vi "azcamtool.vi"() -> ()   [LabVIEW 2014]
doc: "AzCamTool"
uses:
  globals/AzCamGlobals.vi
  globals/DetectorGlobals.vi
panel:
  in  "Image Type":u16(ring) items=["zero", "object", "flat", "dark", "Fe55"]
  in  "Exposure Time":dbl=1.0 min=0.0 format="%<%S%3u>t"
  out "Image Filename":string
  out "StatusBar":string
  in  "TestImage":bool=TRUE caption="Test Image"
  in  "Image Title":string
  out "rowbin":u32=1 min=1 max=99 step=1
  out "colbin":u32=1 min=1 max=99 step=1
  out "progress":dbl(slide) scale=0.0..100.0 scale format="%.1e"
  out "CamTemp":sgl=-999.9 format="%.1f"
  out "DewTemp":sgl=-999.9 format="%.1f"
  out "SequenceCount":string caption="Seq. Count"
  out "Current Exposure Time":dbl caption="Exposure Time" min=0.0 format="%<%S%3u>t"
  out "ImageTypeName":string caption="ImageType"
  in  "Abort":bool
  in  "Reset":bool
  in  "Pause":bool
  in  "Resume":bool
  in  "Readout":bool
  out "CurrentImageTitle":string caption="ImageTitle"
  in  "Expose":bool
  in  "Sequence":bool
  in  "Num Seq.":u16=1 min=1 step=1
  in  "Detector":bool
  in  "FilenameBut":bool caption="Filename"
  in  "Preferences":bool
  out "Test Image":bool
  # "Control"
  # "Status"
  # "Binning"
  # "Exposure Status"
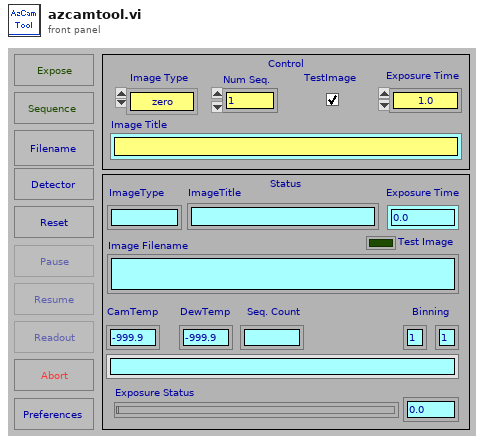
[diagram p1: front panel]
types:
  T1 = enum16{"Standard", "Buffered", "CRLF", "Immediate"}
  T2 = enum16{"Start", "Stop", "Abort", "Pause", "SetExposureTime", "GetExposureTimeRemaining", "Resume", "Readout", "GetExposureTime", "GetTotalPixels", "GetPixelsRemaining"}
  T3 = enum16{"Start", "Stop", "Abort", "Pause", "SetExposureTime", "GetExposureTimeRemaining", "Resume", "Readout", "GetExposureTime"}
  T4 = enum16{"Start", "Stop", "Abort", "Pause", "SetExposureTime", "GetExposureTimeRemaining", "Resume"}
  T5 = enum16{"Start", "Stop", "Abort", "Pause", "SetExposureTime", "GetExposureTimeRemaining", "Resume", "Readout"}
  T6 = enum32{"invalid app kind", "Development System", "Run Time System", "Student Edition", "Embedded LabVIEW", "Evaluation", "Custom"}
  T7 = enum32{"invalid OS target", "Mac OS", "Windows 3.1", "Windows 95/NT", "Solaris 1", "Solaris 2", "HP-UX", "PowerMAX", "Linux", "Irix", "Rhapsody", "BeOS", "AIX", "OSF1", "VxWorks", "PharLap", "Carbon", "RTX", "Windows x64", "Linux x64", "Mac OS X x64"}
  T8 = enum8{"Enabled", "Disabled", "Disabled and Grayed Out"}
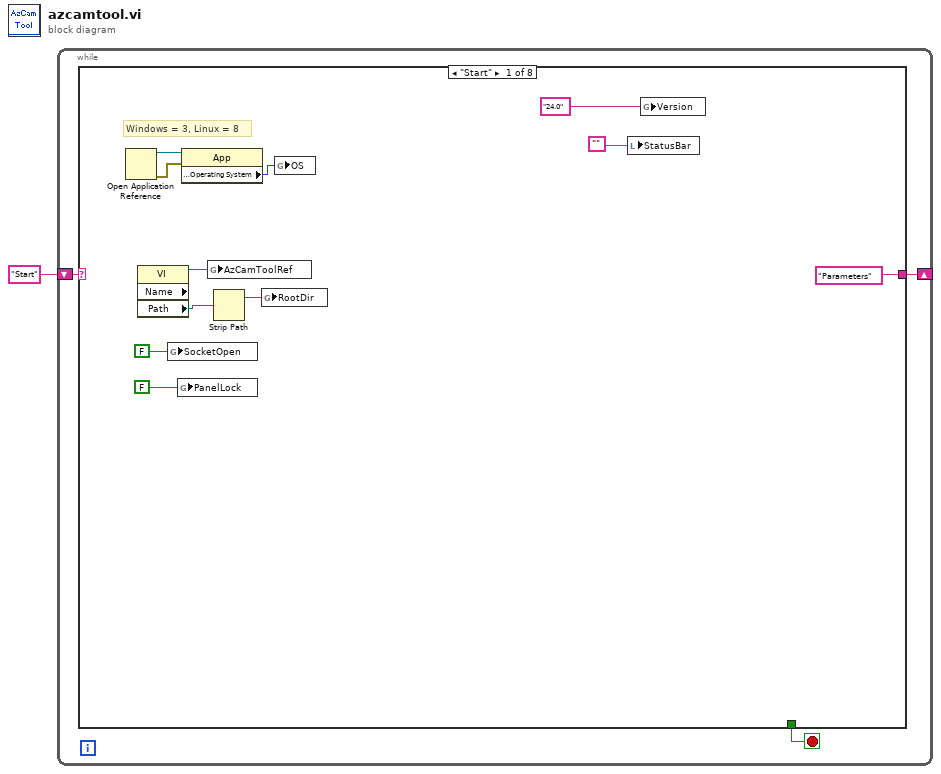
[diagram p0: block diagram]
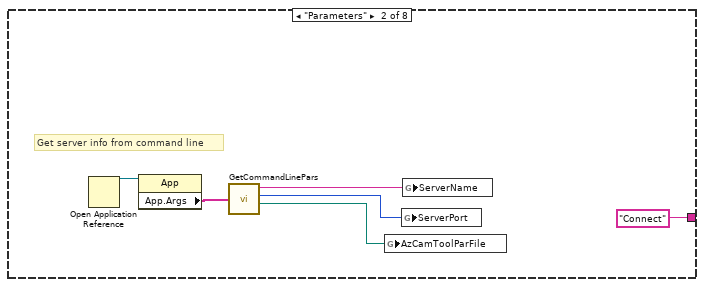
[diagram p2: hidden frame]
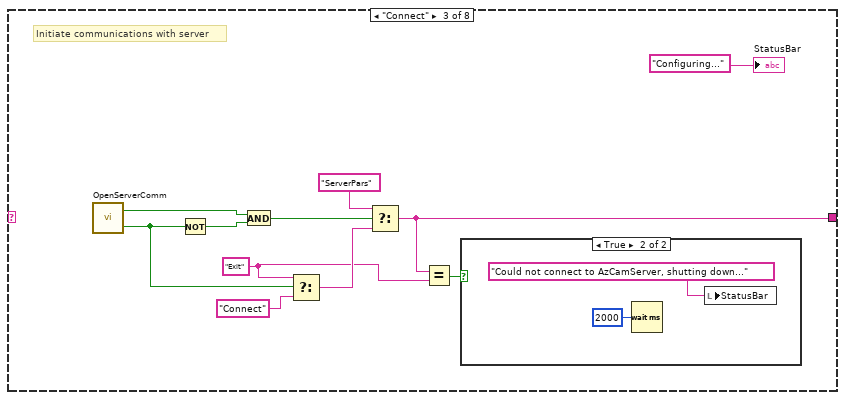
[diagram p3: hidden frame]
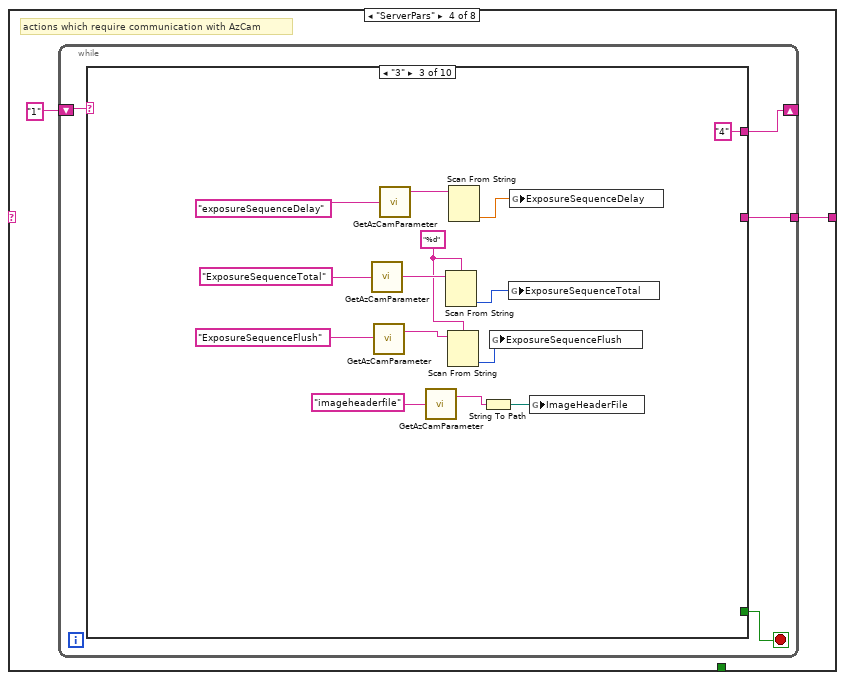
[diagram p5: hidden frame]
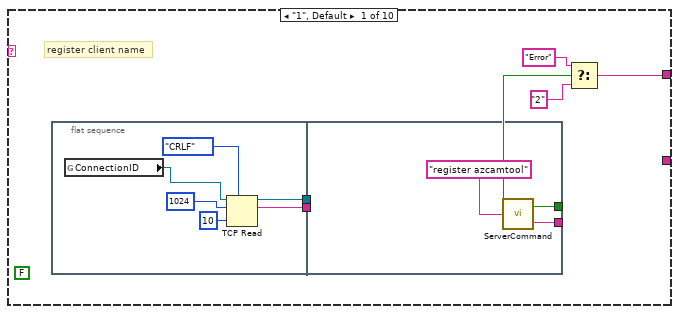
[diagram p6: hidden frame]
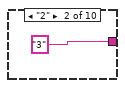
[diagram p7: hidden frame]
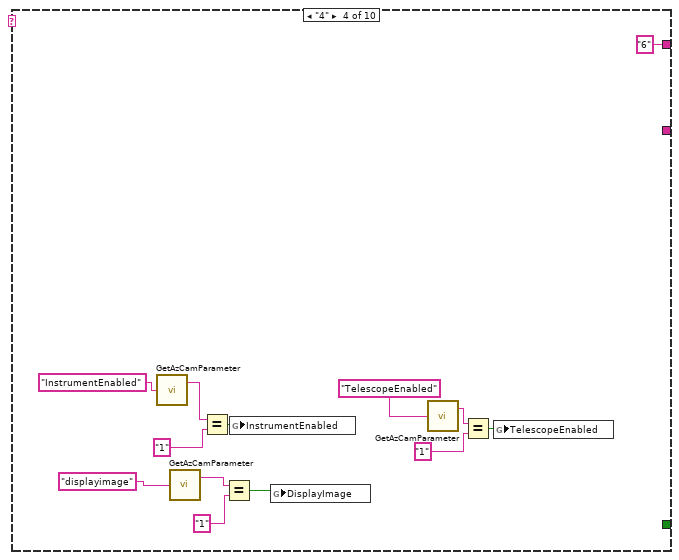
[diagram p8: hidden frame]
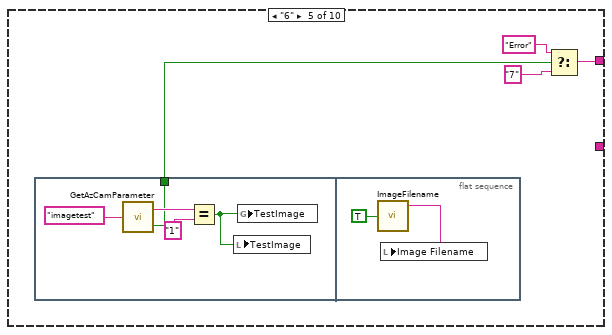
[diagram p9: hidden frame]
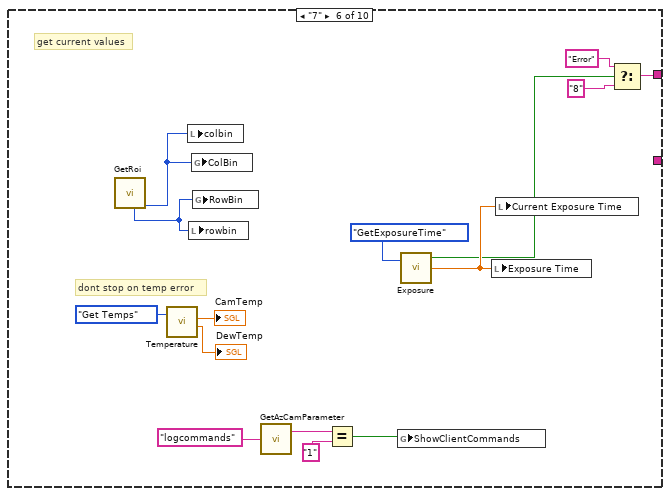
[diagram p10: hidden frame]
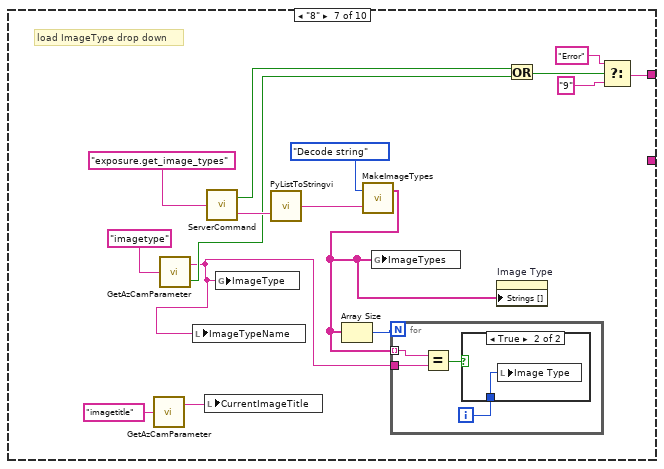
[diagram p11: hidden frame]
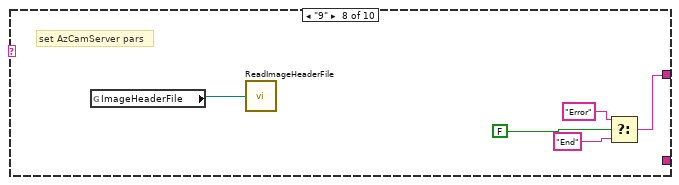
[diagram p13: hidden frame]
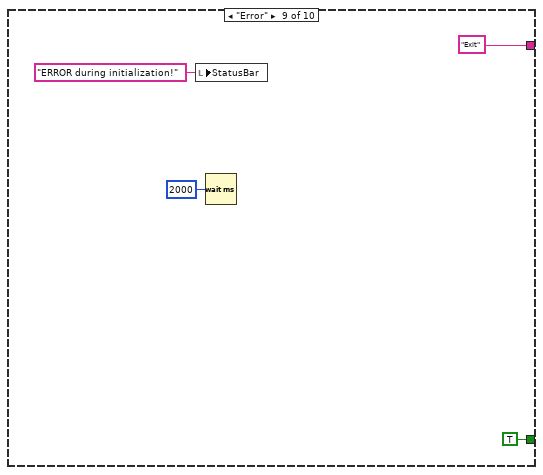
[diagram p14: hidden frame]
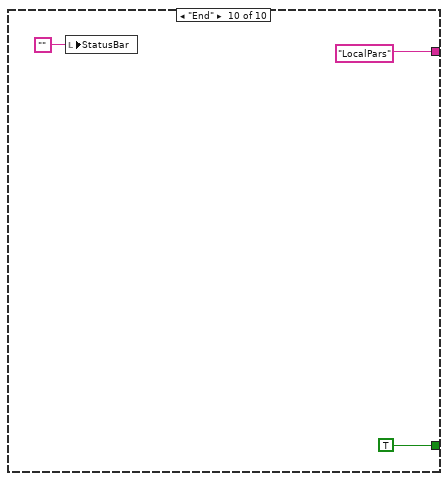
[diagram p15: hidden frame]
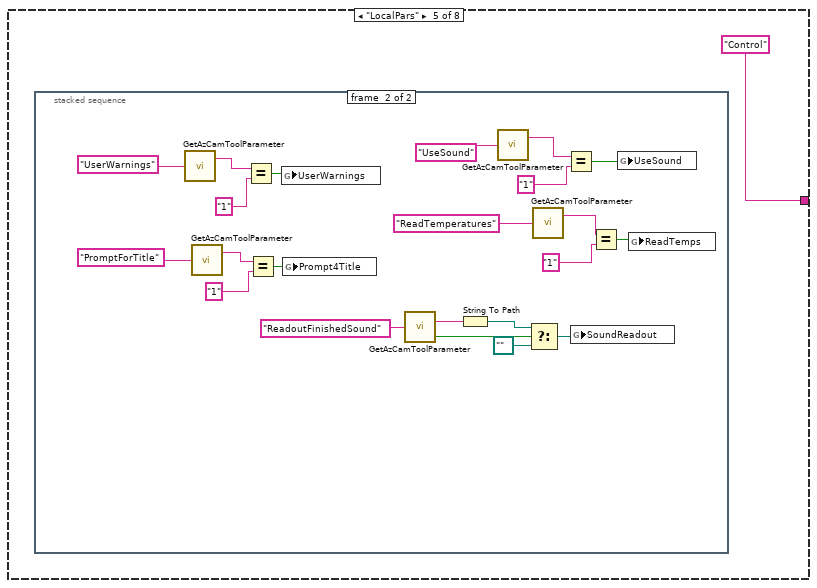
[diagram p16: hidden frame]
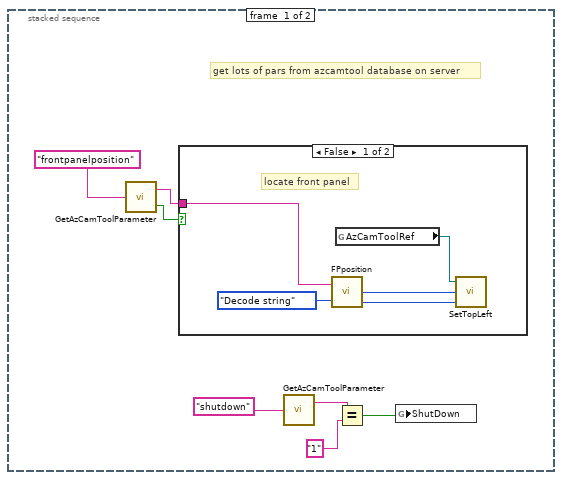
[diagram p17: hidden frame]
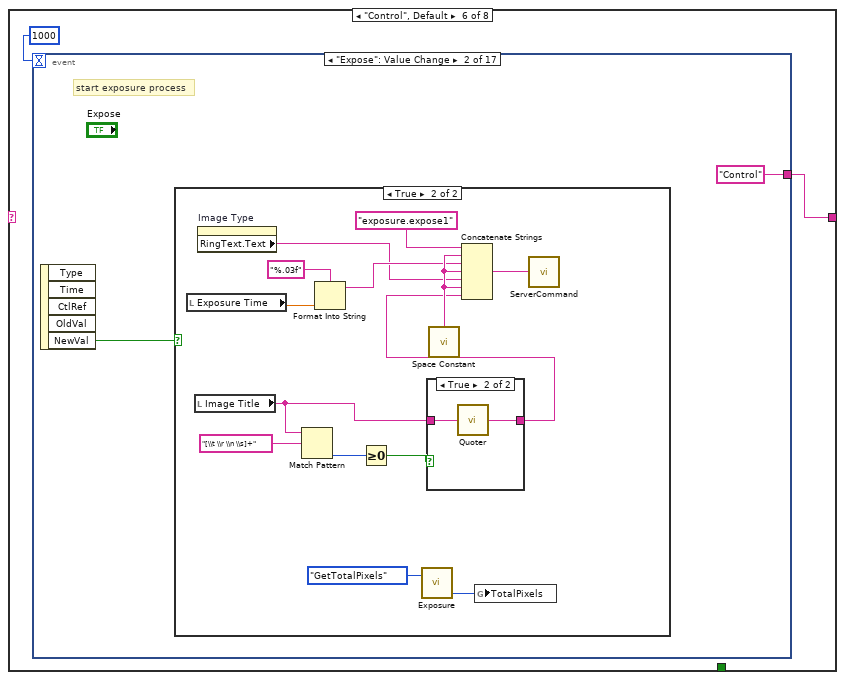
[diagram p19: hidden frame]
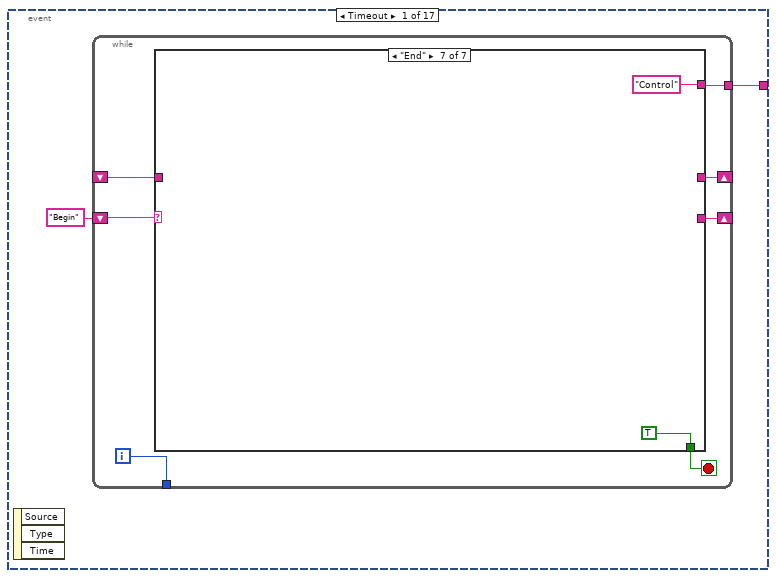
[diagram p20: hidden frame]
diagram:
  n1 = while {
    shift-right: [w2] -> _
    shift-left: "Start" ("Command") -> [w3]
    stop <- w4 stop-if-true
    n2 = case shown="\"Start\"" w3 {
      tunnel: [_ _ _ _ _ _ TRUE TRUE] -> w4
      tunnel: ["Parameters" "Connect" ("f") w24 w36 "Control" w179 _ _] -> w2
      frame "Start" {
        # "Windows = 3, Linux = 8"
        n3 = Open Application Reference() -> (0:w14:errorcluster, 3:w15:refnum<vi>)  [unwired: 4 in]
        n4 = property class="VI" props=["Name", "Path"]() -> (reference out=w6:refnum<vi>, "Path"=w10:path)  [unwired: 2 in, 2 out]
        n5 = global write "AzCamGlobals.vi" "SocketOpen"(FALSE ("SocketOpen")) -> ()
        n6 = global write "AzCamGlobals.vi" "PanelLock"(FALSE ("LockFlag")) -> ()
        n7 = property class="App"(reference=w15, error in=w14) -> ("Application:Target:Operating System"=w12:T7)  [unwired: 2 out]
        n8 = global write "AzCamGlobals.vi" "AzCamToolRef"(w6) -> ()
        n9 = Strip Path(path=w10) -> (stripped path=w8:path)  [unwired: 1 out]
        n10 = global write "AzCamGlobals.vi" "RootDir"(w8) -> ()
        n11 = global write "AzCamGlobals.vi" "OS"(w12) -> ()
        n12 = local write "StatusBar"("") -> ()
        n13 = global write "AzCamGlobals.vi" "Version"("24.0" ("Version Date")) -> ()
      }
      frame "Parameters" {
        # "Get server info from command line"
        n14 = Open Application Reference() -> (3:w19:refnum<vi>)  [unwired: 4 in, 1 out]
        n15 = property class="App"(reference=w19) -> ("App.Args"=w20:string[])  [unwired: 1 in, 2 out]
        n16 = call "GetCommandLinePars.vi"("Command line array"=w20) -> ("Server"=w18:string, "Port"=w17:i32, "AzCamToolParFile"=w16:path)  [unwired: 1 out]
        n17 = global write "AzCamGlobals.vi" "AzCamToolParFile"(w16) -> ()
        n18 = global write "AzCamGlobals.vi" "ServerPort"(w17) -> ()
        n19 = global write "AzCamGlobals.vi" "ServerName"(w18) -> ()
      }
      frame "Connect" {
        w23 = "Exit" ("f")
        # "Initiate communications with server"
        n20 = call "OpenServerComm.vi"() -> ("Connected"=w31:bool, "Quitted"=w25:bool)  [unwired: 1 in]
        n21 = Not(x=w25) -> (.not. x?=w30:bool)
        n22 = And(x=w31, y=w30) -> (x .and. y?=w32:bool)
        n23 = Select(t=w23, s=w25, f="Connect") -> (s? t:f=w27:string)
        n24 = Select(t="ServerPars" ("f"), s=w32, f=w27) -> (s? t:f=w24:string)
        n25 = Equal?(x=w24, y=w23) -> (x = y?=w22:bool)
        n26 = case shown="True" w22 {
          frame False {
          }
          frame True {
            n27 = Wait (ms)(milliseconds to wait=u32 2000) -> ()  [unwired: 1 out]
            n28 = local write "StatusBar"("Could not connect to AzCamServer, shutting down..." ("StatusBar")) -> ()
          }
        }
        "StatusBar" <- "Configuring..." ("Messages")
      }
      frame "ServerPars" {
        # "actions which require communication with AzCam"
        n29 = while {
          tunnel: [w38] -> w36
          shift-right: [w39] -> _
          shift-left: "1" ("key") -> [w40]
          stop <- w37 stop-if-true
          n30 = case shown="\"3\"" w40 {
            tunnel: [w44 "3" ("key") "4" ("key") "6" ("key") w85 w104 w116 w133 _ _] -> w39
            tunnel: [_ _ _ _ _ _ _ _ "Exit" "LocalPars"] -> w38
            tunnel: [_ _ _ _ _ _ _ _ TRUE TRUE] -> w37
            frame "1", Default {
              (unwired) FALSE
              # "register client name"
              n31 = flat-sequence {
                tunnel: [w49] -> w42
                tunnel: [w48] -> w41
                tunnel: [w54] -> _
                tunnel: [w53] -> w43
                tunnel: w42 -> [_]
                tunnel: w41 -> [_]
                frame #0 {
                  n32 = global read "AzCamGlobals.vi" "ConnectionID"() -> (w47:refnum<k5>)
                  n33 = TCP Read(connection ID=w47, bytes to read=1024, 7:T1."CRLF" ("mode (standard)"), 9:10 ("timeout ms (25000)")) -> (connection ID out=w48:refnum<k5>, data out=w49:string)  [unwired: 1 in, 1 out]
                }
                frame #1 {
                  n34 = call "ServerCommand.vi"("Command"="register azcamtool") -> ("Error"=w53:bool, "Reply"=w54:string)
                }
              }
              n35 = Select(t="Error" ("key"), s=w43, f="2" ("key")) -> (s? t:f=w44:string)
            }
            frame "2" {
            }
            frame "3" {
              w65 = "%d" ("format string")
              n36 = call "GetAzCamParameter.vi"("Parameter"="ExposureSequenceTotal") -> ("Value"=w69:string)  [unwired: 1 out]
              n37 = call "GetAzCamParameter.vi"("Parameter"="ExposureSequenceFlush") -> ("Value"=w60:string)  [unwired: 1 out]
              n38 = call "GetAzCamParameter.vi"("Parameter"="exposureSequenceDelay") -> ("Value"=w67:string)  [unwired: 1 out]
              n39 = call "GetAzCamParameter.vi"("Parameter"="imageheaderfile" ("key")) -> ("Value"=w59:string)  [unwired: 1 out]
              n40 = Scan From String(format string=w65, input string=w69) -> (output 1=w63:i32)  [unwired: 3 in, 3 out]
              n41 = Scan From String(format string=w65, input string=w60) -> (output 1=w64:i32)  [unwired: 3 in, 3 out]
              n42 = Scan From String(input string=w67) -> (output 1=w62:dbl)  [unwired: 4 in, 3 out]
              n43 = String To Path(string=w59) -> (path=w61:path)
              n44 = global write "AzCamGlobals.vi" "ExposureSequenceFlush"(w64) -> ()
              n45 = global write "AzCamGlobals.vi" "ExposureSequenceTotal"(w63) -> ()
              n46 = global write "AzCamGlobals.vi" "ExposureSequenceDelay"(w62) -> ()
              n47 = global write "AzCamGlobals.vi" "ImageHeaderFile"(w61) -> ()
            }
            frame "4" {
              n48 = call "GetAzCamParameter.vi"("Parameter"="InstrumentEnabled" ("key")) -> ("Value"=w71:string)  [unwired: 1 out]
              n49 = call "GetAzCamParameter.vi"("Parameter"="displayimage" ("key")) -> ("Value"=w74:string)  [unwired: 1 out]
              n50 = Equal?(x=w71, y="1") -> (x = y?=w79:bool)
              n51 = Equal?(x=w74, y="1") -> (x = y?=w78:bool)
              n52 = global write "AzCamGlobals.vi" "InstrumentEnabled"(w79) -> ()
              n53 = global write "AzCamGlobals.vi" "DisplayImage"(w78) -> ()
              n54 = call "GetAzCamParameter.vi"("Parameter"="TelescopeEnabled" ("key")) -> ("Value"=w75:string)  [unwired: 1 out]
              n55 = Equal?(x=w75, y="1") -> (x = y?=w82:bool)
              n56 = global write "AzCamGlobals.vi" "TelescopeEnabled"(w82) -> ()
            }
            frame "6" {
              n57 = flat-sequence {
                tunnel: [w88] -> w84
                frame #0 {
                  n58 = call "GetAzCamParameter.vi"("Parameter"="imagetest") -> ("Error"=w88:bool, "Value"=w89:string)
                  n59 = Equal?(x=w89, y="1") -> (x = y?=w92:bool)
                  n60 = local write "TestImage"(w92) -> ()
                  n61 = global write "AzCamGlobals.vi" "TestImage"(w92) -> ()
                }
                frame #1 {
                  n62 = call "ImageFilename.vi"("Immediate"=TRUE) -> ("Output Image Filename"=w94:string)  [unwired: 2 out]
                  n63 = local write "Image Filename"(w94) -> ()
                }
              }
              n64 = Select(t="Error" ("key"), s=w84, f="7" ("key")) -> (s? t:f=w85:string)
            }
            frame "7" {
              # "dont stop on temp error"
              # "get current values"
              n65 = call "GetRoi.vi"() -> ("RowBin"=w108:i32, "ColBin"=w109:i32)  [unwired: 1 in, 4 out]
              n66 = call "Temperature.vi"("Action"=enum16{"Set Celsius", "Get Temps"}."Get Temps") -> ("Output2"=→"DewTemp":sgl, "Output1"=→"CamTemp":sgl)  [unwired: 1 in, 3 out]
              n67 = local write "colbin"(w109) -> ()
              n68 = local write "rowbin"(w108) -> ()
              n69 = global write "DetectorGlobals.vi" "ColBin"(w109) -> ()
              n70 = global write "DetectorGlobals.vi" "RowBin"(w108) -> ()
              n71 = call "GetAzCamParameter.vi"("Parameter"="logcommands") -> ("Value"=w96:string)  [unwired: 1 out]
              n72 = Equal?(x=w96, y="1") -> (x = y?=w95:bool)
              n73 = global write "AzCamGlobals.vi" "ShowClientCommands"(w95) -> ()
              n74 = call "Exposure.vi"("Command"=T2."GetExposureTime") -> ("Error"=w99:bool, "float"=w100:dbl)  [unwired: 1 in, 1 out]
              n75 = local write "Exposure Time"(w100) -> ()
              n76 = local write "Current Exposure Time"(w100) -> ()
              n77 = Select(t="Error" ("key"), s=w99, f="8" ("key")) -> (s? t:f=w104:string)
            }
            frame "8" {
              # "load ImageType drop down"
              n78 = call "GetAzCamParameter.vi"("Parameter"="imagetitle") -> ("Value"=w110:string)  [unwired: 1 out]
              n79 = call "GetAzCamParameter.vi"("Parameter"="imagetype") -> ("Error"=w113:bool, "Value"=w112:string)
              n80 = local write "ImageTypeName"(w112) -> ()
              n81 = local write "CurrentImageTitle"(w110) -> ()
              n82 = call "ServerCommand.vi"("Command"="exposure.get_image_types") -> ("Error"=w114:bool, "Reply"=w123:string)
              n83 = global write "AzCamGlobals.vi" "ImageType"(w112) -> ()
              n84 = call "PyListToStringvi.vi"("PythonList"=w123) -> ("String"=w122:string)
              n85 = call "MakeImageTypes.vi"("String In"=w122, "Action"=enum16{"Make string", "Decode string"}."Decode string") -> ("ImageTypes"=w120:string[])  [unwired: 1 out]
              n86 = Array Size(array=w120) -> (size(s)=w121:i32)
              n87 = global write "AzCamGlobals.vi" "ImageTypes"(w120) -> ()
              n88 = for {
                N: w121 -> [_]
                tunnel: w120 -> [w129] mode=indexing
                tunnel: w112 -> [w128]
                i -> [w126]
                n89 = Equal?(x=w129, y=w128) -> (x = y?=w127:bool)
                n90 = case shown="True" w127 {
                  tunnel: w126 -> [_ w130]
                  frame False {
                  }
                  frame True {
                    n91 = local write "Image Type"(w130) -> ()
                  }
                }
              }
              n92 = property on="Image Type" class="Ring (strict)"("Strings []"=w120) -> ()  [unwired: 2 in, 2 out]
              n93 = Or(x=w114, y=w113) -> (x .or. y?=w115:bool)
              n94 = Select(t="Error" ("key"), s=w115, f="9" ("key")) -> (s? t:f=w116:string)
            }
            frame "9" {
              # "set AzCamServer pars"
              n95 = global read "AzCamGlobals.vi" "ImageHeaderFile"() -> (w132:path)
              n96 = call "ReadImageHeaderFile.vi"("ImageHeaderFile"=w132) -> ()  [unwired: 1 in]
              n97 = Select(t="Error" ("key"), s=FALSE, f="End" ("key")) -> (s? t:f=w133:string)
            }
            frame "Error" {
              n98 = local write "StatusBar"("ERROR during initialization!" ("StatusBar")) -> ()
              n99 = Wait (ms)(milliseconds to wait=u32 2000) -> ()  [unwired: 1 out]
            }
            frame "End" {
              n100 = local write "StatusBar"("") -> ()
            }
          }
        }
      }
      frame "LocalPars" {
        n101 = stacked-sequence {
          frame #0 {
            # "get lots of pars from azcamtool database on server"
            n102 = call "GetAzCamToolParameter.vi"("Parameter"="frontpanelposition" ("key")) -> ("Error"=w149:bool, "Value"=w150:string)
            n103 = case shown="False" w149 {
              tunnel: w150 -> [w151 _]
              frame False {
                # "locate front panel"
                n104 = call "FPposition.vi"("String In"=w151, "Action"=enum16{"Make string", "Decode string"}."Decode string") -> ("top"=w153:i32, "left"=w152:i32)  [unwired: 1 out]
                n105 = global read "AzCamGlobals.vi" "AzCamToolRef"() -> (w155:refnum<vi>)
                n106 = call "SetTopLeft.vi"("left"=w152, "top"=w153, "VI Ref"=w155) -> ()
              }
              frame True {
              }
            }
            n107 = call "GetAzCamToolParameter.vi"("Parameter"="shutdown" ("key")) -> ("Value"=w144:string)  [unwired: 1 out]
            n108 = Equal?(x=w144, y="1") -> (x = y?=w147:bool)
            n109 = global write "AzCamGlobals.vi" "ShutDown"(w147) -> ()
          }
          frame #1 {
            n110 = call "GetAzCamToolParameter.vi"("Parameter"="UserWarnings" ("key")) -> ("Value"=w158:string)  [unwired: 1 out]
            n111 = call "GetAzCamToolParameter.vi"("Parameter"="PromptForTitle" ("key")) -> ("Value"=w159:string)  [unwired: 1 out]
            n112 = Equal?(x=w158, y="1") -> (x = y?=w176:bool)
            n113 = Equal?(x=w159, y="1") -> (x = y?=w174:bool)
            n114 = global write "AzCamGlobals.vi" "UserWarnings"(w176) -> ()
            n115 = global write "AzCamGlobals.vi" "Prompt4Title"(w174) -> ()
            n116 = call "GetAzCamToolParameter.vi"("Parameter"="ReadoutFinishedSound" ("key")) -> ("Error"=w156:bool, "Value"=w160:string)
            n117 = String To Path(string=w160) -> (path=w168:path)
            n118 = call "GetAzCamToolParameter.vi"("Parameter"="UseSound" ("key")) -> ("Value"=w177:string)  [unwired: 1 out]
            n119 = Select(t=w168, s=w156, f=path "") -> (s? t:f=w170:path)
            n120 = call "GetAzCamToolParameter.vi"("Parameter"="ReadTemperatures" ("key")) -> ("Value"=w165:string)  [unwired: 1 out]
            n121 = Equal?(x=w177, y="1") -> (x = y?=w171:bool)
            n122 = global write "AzCamGlobals.vi" "SoundReadout"(w170) -> ()
            n123 = Equal?(x=w165, y="1") -> (x = y?=w167:bool)
            n124 = global write "AzCamGlobals.vi" "UseSound"(w171) -> ()
            n125 = global write "AzCamGlobals.vi" "ReadTemps"(w167) -> ()
          }
        }
      }
      frame "Control", Default {
        n126 = event shown="[1] \"Expose\": Value Change" {
          selector: _ -> [_ _ _ _ _ _ _ _ _ _ _ _ _ _ _ _ _]
          dyn-events: _ -> [_ _ _ _ _ _ _ _ _ _ _ _ _ _ _ _ _]
          timeout: 1000 -> [_ _ _ _ _ _ _ _ _ _ _ _ _ _ _ _ _]
          tunnel: [w181 "Control" ("Command") "Control" ("Command") _ _ _ _ _ _ _ _ _ _ _ _ "Exit" ("Command") w408] -> w179
          event Timeout {
            n127 = event-data() -> ()  [unwired: 1 in, 3 out]
            n128 = while {
              shift-right: [w187] -> _
              shift-left: "Begin" -> [w188]
              tunnel: [w186] -> w181
              tunnel: [w185] -> _
              shift-right: [w184] -> _
              shift-left: _ -> [w183]
              i -> [w185]
              stop <- w182 stop-if-true
              n129 = case shown="\"End\"" w188 {
                tunnel: [w191 "Pars" "TimeSync" "CheckExposing" w249 "End" _] -> w187
                tunnel: [w189 _ w216 w238 w247 _ TRUE ("Error")] -> w182
                tunnel: [w190 _ _ _ _ _ "Control"] -> w186
                tunnel: [_ _ _ _ w252 _ _] -> w184
                tunnel: w183 -> [_ _ _ _ _ w276 _]
                frame "Begin", Default {
                  n130 = global read "AzCamGlobals.vi" "SocketOpen"() -> (w192:bool)
                  n131 = case shown="False" w192 {
                    tunnel: [_ "Temps"] -> w191
                    tunnel: ["Quit" ("f") _] -> w190
                    tunnel: [TRUE FALSE] -> w189
                    frame False {
                      n132 = local write "StatusBar"("No communication with AzCamServer..." ("message")) -> ()
                      n133 = Wait (ms)(milliseconds to wait=u32 1000) -> ()  [unwired: 1 out]
                    }
                    frame True {
                    }
                  }
                }
                frame "Temps" {
                  # "update status on timeout only..."
                  n134 = flat-sequence {
                    frame #0 {
                      n135 = call "Temperature.vi"("Action"=enum16{"Set Celsius", "Get Temps"}."Get Temps") -> ("Output2"=w200:sgl, "Output1"=w201:sgl)  [unwired: 1 in, 3 out]
                      n136 = local write "CamTemp"(w201) -> ()
                      n137 = local write "DewTemp"(w200) -> ()
                    }
                    frame #1 {
                      n138 = call "GetAzCamParameter.vi"("Parameter"="imagetitle" ("Attribute")) -> ("Error"=w204:bool, "Value"=w208:string)
                      n139 = call "GetAzCamParameter.vi"("Parameter"="imagetest" ("Attribute")) -> ("Error"=w203:bool, "Value"=w205:string)
                      n140 = case shown="False" w203 {
                        tunnel: w205 -> [w211 _]
                        frame False {
                          n141 = Equal?(x=w211, y="1") -> (x = y?=→"Test Image":bool)
                        }
                        frame True {
                        }
                      }
                      n142 = case shown="False" w204 {
                        tunnel: w208 -> [w212 _]
                        frame False {
                          "CurrentImageTitle" <- w212
                        }
                        frame True {
                        }
                      }
                    }
                  }
                }
                frame "Pars" {
                  n143 = call "GetBoolean.vi"("Attribute"="isexposuresequence") -> ("Error"=w215:bool, "Boolean"=w213:bool)
                  n144 = case shown="False" w213 {
                    tunnel: [_ w229] -> w218
                    tunnel: [_ w231] -> w217
                    tunnel: ["" w225] -> w214
                    frame False {
                    }
                    frame True {
                      n145 = call "GetAzCamParameter.vi"("Parameter"="exposuresequencenumber" ("Attribute")) -> ("Error"=w231:bool, "Value"=w228:string)
                      n146 = call "GetAzCamParameter.vi"("Parameter"="exposuresequencetotal" ("Attribute")) -> ("Error"=w229:bool, "Value"=w227:string)
                      n147 = Concatenate Strings(w228, "/" ("string"), w227) -> (w225:string)
                    }
                  }
                  "SequenceCount" <- w214
                  n148 = call "Exposure.vi"("Command"=T2."GetExposureTime") -> ("Error"=w219:bool, "float"=w221:dbl)  [unwired: 1 in, 1 out]
                  n149 = local write "Sequence"(w213) -> ()
                  n150 = case shown="True" w219 {
                    tunnel: w221 -> [w233 _]
                    frame False {
                      n151 = call "GetRoi.vi"() -> ("RowBin"=w235:i32, "ColBin"=w234:i32)  [unwired: 1 in, 4 out]
                      "rowbin" <- w235
                      "colbin" <- w234
                      n152 = global write "DetectorGlobals.vi" "ColBin"(w234) -> ()
                      n153 = global write "DetectorGlobals.vi" "RowBin"(w235) -> ()
                      "Current Exposure Time" <- w233
                    }
                    frame True {
                    }
                  }
                  n154 = Compound Arithmetic op=OR(w217, w218, w215, w219) -> (w216:bool)
                }
                frame "TimeSync" {
                  n155 = call "GetBoolean.vi"("Attribute"="exposurecompleted") -> ("Error"=w238:bool, "Boolean"=w239:bool)
                  n156 = call "ImageFilename.vi"("Immediate"=TRUE) -> ("Output Image Filename"=w237:string)  [unwired: 2 out]
                  n157 = case shown="True" w239 {
                    frame False {
                    }
                    frame True {
                      n158 = global read "AzCamGlobals.vi" "UseSound"() -> (w242:bool)
                      n159 = case shown="True" w242 {
                        frame False {
                        }
                        frame True {
                          n160 = global read "AzCamGlobals.vi" "SoundReadout"() -> (w243:path)
                          n161 = call "sound.vi"("Sound File"=w243) -> ()
                        }
                      }
                    }
                  }
                  n162 = local write "Image Filename"(w237) -> ()
                }
                frame "CheckExposing" {
                  n163 = call "GetAzCamParameter.vi"("Parameter"="exposureflag") -> ("Error"=w247:bool, "Value"=w246:string)
                  n164 = case shown="True" w247 {
                    tunnel: w246 -> [w272 _]
                    tunnel: [w270 w273] -> w253
                    tunnel: [w271 ""] -> w252
                    frame False {
                      n165 = call "ExposureStatusMessage.vi"("ExposureFlag"=w272) -> ("Message"=w271:string, "Exposing"=w270:bool)
                      n166 = local write "Expose"(w270) -> ()
                    }
                    frame True {
                      w273 = FALSE ("Exposing")
                      n167 = local write "Expose"(w273) -> ()
                    }
                  }
                  n168 = case shown="True" w253 {
                    tunnel: ["End" "Exposing"] -> w249
                    tunnel: w252 -> [_ w264]
                    tunnel: [w255 w267] -> w251
                    tunnel: [w255 w265] -> w250
                    frame False {
                      w255 = T8."Disabled and Grayed Out" ("Disabled")
                      n169 = local write "StatusBar"("") -> ()
                      n170 = local write "Pause"(FALSE ("Pause")) -> ()
                      "progress" <- 0.0 ("progress")
                    }
                    frame True {
                      w262 = T8."Enabled" ("Disabled")
                      w266 = T8."Disabled and Grayed Out" ("Disabled")
                      n171 = Equal?(x=w264, y="Exposure paused" ("Message")) -> (x = y?=w260:bool)
                      n172 = local write "StatusBar"(w264) -> ()
                      n173 = Equal?(x=w264, y="Reading image" ("Message")) -> (x = y?=w261:bool)
                      n174 = Or(x=w260, y=w261) -> (x .or. y?=w259:bool)
                      n175 = Select(t=w262, s=w260, f=w266) -> (s? t:f=w267:T8)
                      n176 = Select(t=w266, s=w259, f=w262) -> (s? t:f=w265:T8)
                    }
                  }
                  n177 = property on="Readout" class="Bool"("DisabledEnum"=w251) -> ()  [unwired: 2 in, 2 out]
                  n178 = property on="Resume" class="Bool"("DisabledEnum"=w251) -> ()  [unwired: 2 in, 2 out]
                  n179 = property on="Pause" class="Bool (strict)"("DisabledEnum"=w250) -> ()  [unwired: 2 in, 2 out]
                  n180 = call "GetAzCamParameter.vi"("Parameter"="imagetype") -> ("Value"=→"ImageTypeName":string)  [unwired: 1 out]
                }
                frame "Exposing" {
                  n181 = case shown="Default" w276 {
                    selector: w276 -> [_ w284 w290 w299 w302]
                    frame Default {
                      n182 = property on="progress" class="Slide (strict)"("Scale.Maximum"=100.0 ("Scale.Range:Maximum"), "Scale.Minimum"=0.0 ("Scale.Range:Minimum"), "Value"=0.0 ("progress")) -> ()  [unwired: 2 in, 2 out]
                    }
                    frame "Exposing" {
                      n183 = local write "StatusBar"(w284) -> ()
                      n184 = call "Exposure.vi"("Command"=T3."GetExposureTimeRemaining") -> ("float"=w282:dbl)  [unwired: 1 in, 2 out]
                      n185 = call "Exposure.vi"("Command"=T2."GetExposureTime") -> ("float"=w280:dbl)  [unwired: 1 in, 2 out]
                      n186 = property on="progress" class="Slide (strict)"("Scale.Maximum"=w280, "Scale.Minimum"=0.0 ("Scale.Range:Minimum"), "Value"=w282) -> ()  [unwired: 2 in, 2 out]
                    }
                    frame "Exposure paused" {
                      n187 = local write "StatusBar"(w290) -> ()
                      n188 = call "Exposure.vi"("Command"=T3."GetExposureTimeRemaining") -> ("float"=w288:dbl)  [unwired: 1 in, 2 out]
                      n189 = call "Exposure.vi"("Command"=T2."GetExposureTime") -> ("float"=w286:dbl)  [unwired: 1 in, 2 out]
                      n190 = property on="progress" class="Slide (strict)"("Scale.Maximum"=w286, "Scale.Minimum"=0.0 ("Scale.Range:Minimum"), "Value"=w288) -> ()  [unwired: 2 in, 2 out]
                    }
                    frame "Reading image" {
                      n191 = local write "StatusBar"(w299) -> ()
                      n192 = call "Exposure.vi"("Command"=T2."GetTotalPixels") -> ("integer"=w292:i32)  [unwired: 1 in, 2 out]
                      n193 = call "Exposure.vi"("Command"=T2."GetPixelsRemaining") -> ("integer"=w295:i32)  [unwired: 1 in, 2 out]
                      n194 = Divide(x=w295, y=w292) -> (x/y=w298:dbl)
                      n195 = Multiply(x=w298, y=100.0) -> (x*y=w294:dbl)
                      n196 = property on="progress" class="Slide (strict)"("Scale.Maximum"=100.0 ("Scale.Range:Maximum"), "Scale.Minimum"=0.0 ("Scale.Range:Minimum"), "Value"=w294) -> ()  [unwired: 2 in, 2 out]
                    }
                    frame "Image Writing" {
                      n197 = local write "StatusBar"(w302) -> ()
                      n198 = local write "progress"(0.0 ("progress")) -> ()
                    }
                  }
                }
                frame "End" {
                }
              }
            }
          }
          event "Expose": Value Change {
            # "start exposure process"
            n199 = event-data() -> ("NewVal"=w307:bool)  [unwired: 1 in, 4 out]
            n200 = case shown="True" w307 {
              frame False {
              }
              frame True {
                n201 = local read "Exposure Time"() -> (w320:dbl)
                n202 = local read "Image Title"() -> (w309:string)
                n203 = property on="Image Type" class="Ring (strict)"() -> ("RingText.Text"=w315:string)  [unwired: 2 in, 2 out]
                n204 = Match Pattern(string=w309, regular expression="[\\t \\r \\n \\s]+") -> (offset past match=w312:i32)  [unwired: 1 in, 3 out]
                n205 = Format Into String(format string="%.03f", w320) -> (resulting string=w316:string)  [unwired: 2 in, 1 out]
                n206 = Greater Or Equal To 0?(x=w312) -> (x >= 0?=w310:bool)
                n207 = call "Exposure.vi"("Command"=T2."GetTotalPixels") -> ("integer"=w313:i32)  [unwired: 1 in, 2 out]
                n208 = case shown="True" w310 {
                  tunnel: [w322 w324] -> w308
                  tunnel: w309 -> [w322 w323]
                  frame False {
                  }
                  frame True {
                    n209 = call "Quoter.vi"("String In"=w323) -> ("String Out"=w324:string)
                  }
                }
                n210 = call <vilib>:"Space Constant.vi"() -> ("String"=w318:string)
                n211 = Concatenate Strings("exposure.expose1", w318, w316, w318, w315, w318, w308) -> (w317:string)
                n212 = global write "AzCamGlobals.vi" "TotalPixels"(w313) -> ()
                n213 = call "ServerCommand.vi"("Command"=w317) -> ()  [unwired: 2 out]
              }
            }
          }
          event "Sequence": Value Change {
            n214 = event-data() -> ("OldVal"=w326:bool, "NewVal"=w325:bool)  [unwired: 1 in, 4 out]
            n215 = local read "Expose"() -> (w329:bool)
            n216 = Not(x=w329) -> (.not. x?=w328:bool)
            n217 = Compound Arithmetic op=AND(w325, w328) -> (w330:bool)
            n218 = case shown="True" w330 {
              tunnel: w326 -> [w332 _]
              tunnel: w325 -> [w334 _]
              frame False {
                n219 = Not(x=w334) -> (.not. x?=w333:bool)
                n220 = Compound Arithmetic op=AND(w332, w333) -> (w331:bool)
                n221 = case shown="True" w331 {
                  frame False {
                  }
                  frame True {
                    n222 = stacked-sequence {
                      frame #0 {
                        n223 = local write "StatusBar"("stopping exposure sequence..." ("StatusBar")) -> ()
                      }
                      frame #1 {
                        n224 = call "SetAzCamParameter.vi"("Value"="0", "Parameter"="isexposuresequence" ("Command")) -> ()  [unwired: 1 out]
                        n225 = call "SetAzCamParameter.vi"("Value"="1", "Parameter"="exposuresequencetotal" ("Attribute")) -> ()  [unwired: 1 out]
                      }
                    }
                  }
                }
              }
              frame True {
                n226 = local read "Test Image"() -> (w341:bool)
                n227 = global read "AzCamGlobals.vi" "UserWarnings"() -> (w342:bool)
                n228 = And(x=w342, y=w341) -> (x .and. y?=w340:bool)
                n229 = case shown="True" w340 {
                  tunnel: [TRUE ("T button?") w345] -> w343
                  frame False {
                  }
                  frame True {
                    n230 = Two Button Dialog(message="Do you really want to take a sequence of test exposures?", 2:"Yes" ("button name (\"OK\")")) -> (T button?=w345:bool)  [unwired: 1 in]
                  }
                }
                n231 = case shown="True" w343 {
                  frame False {
                  }
                  frame True {
                    n232 = stacked-sequence {
                      frame #0 {
                        n233 = local read "Exposure Time"() -> (w348:dbl)
                        n234 = call "Exposure.vi"("Command"=T2."SetExposureTime", "Exposure Time"=w348) -> ()  [unwired: 3 out]
                      }
                      frame #1 {
                        n235 = property on="Image Type" class="Ring (strict)"() -> ("RingText.Text"=w350:string)  [unwired: 2 in, 2 out]
                        n236 = call "ImageType.vi"("ImageType"=w350) -> ()  [unwired: 4 out]
                      }
                      frame #2 {
                        n237 = global read "AzCamGlobals.vi" "ExposureSequenceDelay"() -> (w351:dbl)
                        n238 = Format Into String(w351) -> (resulting string=w353:string)  [unwired: 3 in, 1 out]
                        n239 = call "SetAzCamParameter.vi"("Value"=w353, "Parameter"="exposuresequencedelay" ("string")) -> ()  [unwired: 1 out]
                      }
                      frame #3 {
                        n240 = call "Exposure.vi"("Command"=T2."GetTotalPixels") -> ("integer"=w354:i32)  [unwired: 1 in, 2 out]
                        n241 = global write "AzCamGlobals.vi" "TotalPixels"(w354) -> ()
                      }
                      frame #4 {
                        n242 = Format Into String("Num Seq.") -> (resulting string=w359:string)  [unwired: 3 in, 1 out]
                        n243 = call <vilib>:"Space Constant.vi"() -> ("String"=w357:string)
                        n244 = Concatenate Strings("exposure.sequence1 " ("Command"), w359, w357, "-1") -> (w358:string)
                        n245 = call "ServerCommand.vi"("Command"=w358) -> ()  [unwired: 2 out]
                      }
                    }
                  }
                }
              }
            }
          }
          event "Detector": Value Change {
            n246 = event-data() -> ()  [unwired: 1 in, 6 out]
            n247 = flat-sequence {
              frame #0 {
                n248 = call "DetPars.vi"("Immediate"=FALSE) -> ()  [unwired: 1 out]
              }
              frame #1 {
                n249 = global read "DetectorGlobals.vi" "ColBin"() -> (w364:i32)
                n250 = global read "DetectorGlobals.vi" "RowBin"() -> (w363:i32)
                n251 = local write "rowbin"(w363) -> ()
                n252 = local write "colbin"(w364) -> ()
              }
              frame #2 {
              }
              frame #3 {
                n253 = call "SavePars.vi"() -> ()  [unwired: 1 in, 1 out]
              }
            }
          }
          event "Preferences": Value Change {
            n254 = event-data() -> ()  [unwired: 1 in, 6 out]
            n255 = stacked-sequence {
              frame #0 {
                n256 = call "Preferences.vi"() -> ()  [unwired: 1 in]
              }
              frame #1 {
                n257 = call "SavePars.vi"() -> ()  [unwired: 1 in, 1 out]
              }
            }
          }
          event "Reset": Value Change {
            n258 = event-data() -> ()  [unwired: 1 in, 5 out]
            n259 = flat-sequence {
              frame #0 {
                n260 = call "ResetController.vi"() -> ()  [unwired: 2 in, 1 out]
              }
              frame #1 {
              }
            }
          }
          event "FilenameBut": Value Change {
            n261 = event-data() -> ()  [unwired: 1 in, 5 out]
            n262 = flat-sequence {
              frame #0 {
                n263 = call "ImageFilename.vi"("Immediate"=FALSE) -> ("Output Image Filename"=w366:string, "TestImage"=w368:bool, "Error"=w365:bool)
                n264 = case shown="False" w365 {
                  tunnel: w368 -> [w370 _]
                  tunnel: w366 -> [w369 _]
                  frame False {
                    n265 = local write "TestImage"(w370) -> ()
                    n266 = call "SavePars.vi"() -> ()  [unwired: 1 in, 1 out]
                    "Image Filename" <- w369
                  }
                  frame True {
                  }
                }
              }
              frame #1 {
              }
            }
          }
          event "TestImage": Value Change {
            n267 = event-data() -> ()  [unwired: 1 in, 6 out]
            n268 = flat-sequence {
              frame #0 {
                n269 = Select(t="1", s="TestImage", f="0") -> (s? t:f=w371:string)
                n270 = global write "AzCamGlobals.vi" "TestImage"("TestImage") -> ()
                n271 = call "SetAzCamParameter.vi"("Value"=w371, "Parameter"="imagetest") -> ()  [unwired: 1 out]
              }
              frame #1 {
                n272 = call "ImageFilename.vi"("Immediate"=TRUE) -> ("Output Image Filename"=w377:string)  [unwired: 2 out]
                n273 = local write "Image Filename"(w377) -> ()
              }
            }
          }
          event "Image Type": Value Change {
            n274 = event-data() -> ()  [unwired: 1 in, 6 out]
            n275 = property on="Image Type" class="Ring (strict)"() -> ("RingText.Text"=w378:string)  [unwired: 2 in, 2 out]
            n276 = call "ImageType.vi"("ImageType"=w378) -> ()  [unwired: 4 out]
          }
          event "Image Title": Value Change {
            n277 = event-data() -> ()  [unwired: 1 in, 6 out]
            n278 = Match Pattern(string="Image Title", regular expression="[\\t \\r \\n \\s]+") -> (offset past match=w381:i32)  [unwired: 1 in, 3 out]
            n279 = Greater Or Equal To 0?(x=w381) -> (x >= 0?=w380:bool)
            n280 = case shown="True" w380 {
              tunnel: [w385 w387] -> w383
              tunnel: "Image Title" -> [w385 w386]
              frame False {
              }
              frame True {
                n281 = call "Quoter.vi"("String In"=w386) -> ("String Out"=w387:string)
              }
            }
            n282 = call "SetAzCamParameter.vi"("Value"=w383, "Parameter"="imagetitle ") -> ()  [unwired: 1 out]
          }
          event "Exposure Time": Value Change {
            n283 = event-data() -> ("NewVal"=w389:dbl)  [unwired: 1 in, 5 out]
            n284 = call "Exposure.vi"("Command"=T2."SetExposureTime", "Exposure Time"=w389) -> ()  [unwired: 3 out]
          }
          event "Abort": Value Change {
            n285 = event-data() -> ()  [unwired: 1 in, 6 out]
            n286 = call "Exposure.vi"("Command"=T2."Abort") -> ("Error"=w390:bool)  [unwired: 1 in, 2 out]
            n287 = stacked-sequence {
              tunnel: w390 -> [_]
              frame #0 {
                n288 = local read "Sequence"() -> (w393:bool)
                n289 = local write "Abort"(FALSE ("Abort")) -> ()
                n290 = case shown="True" w393 {
                  frame False {
                    n291 = local write "progress"(0.0 ("progress")) -> ()
                  }
                  frame True {
                    n292 = Wait (ms)(milliseconds to wait=u32 1000) -> ()  [unwired: 1 out]
                    n293 = local write "StatusBar"("aborting sequence and current exposure" ("StatusBar")) -> ()
                  }
                }
              }
            }
          }
          event "Pause": Value Change {
            n294 = event-data() -> ("NewVal"=w397:bool)  [unwired: 1 in, 5 out]
            n295 = case shown="True" w397 {
              frame False {
              }
              frame True {
                n296 = call "Exposure.vi"("Command"=T4."Pause") -> ()  [unwired: 1 in, 3 out]
              }
            }
          }
          event "Readout": Value Change {
            n297 = event-data() -> ()  [unwired: 1 in, 6 out]
            n298 = call "Exposure.vi"("Command"=T5."Readout") -> ()  [unwired: 1 in, 3 out]
          }
          event "Resume": Value Change {
            n299 = event-data() -> ()  [unwired: 1 in, 6 out]
            n300 = call "Exposure.vi"("Command"=T5."Resume") -> ("Error"=w400:bool)  [unwired: 1 in, 2 out]
            n301 = stacked-sequence {
              tunnel: w400 -> [_]
              frame #0 {
                n302 = local write "Pause"(FALSE ("Pause")) -> ()
              }
            }
          }
          event Panel Close {
            n303 = event-data() -> ()  [unwired: 1 in, 4 out]
            n304 = One Button Dialog(message="close") -> ()  [unwired: 1 in, 1 out]
          }
          event Menu Selection (User) {
            n305 = event-data() -> ("MenuRef"=w407:refnum<k9>, "ItemTag"=w406:string, "ItemPath"=w405:string)  [unwired: 1 in, 4 out]
            n306 = call "MenuFind.vi"("TagIn"=w405) -> ("Menu"=w409:string)
            n307 = case shown="\"Help\"" w409 {
              tunnel: w407 -> [_ _ w413]
              tunnel: [_ w411 _] -> w408
              tunnel: w406 -> [_ w410 w414]
              frame Default {
              }
              frame "File" {
                n308 = case shown="\"Exit\"" w410 {
                  tunnel: [_ "Exit" ("Command")] -> w411
                  frame Default {
                  }
                  frame "Exit" {
                  }
                }
              }
              frame "Help" {
                n309 = case shown="\"AboutAzCam\"" w414 {
                  selector: w414 -> [_ w417 _]
                  tunnel: w413 -> [_ w415 _]
                  frame Default {
                  }
                  frame "DisplayTips" {
                    n310 = call "MenuToggle.vi"("item tag"=w417, "menubar"=w415) -> ("checked"=w416:bool)
                    n311 = property class="App"("Application:Show FP Tip Strips"=w416) -> ()  [unwired: 2 in, 2 out]
                  }
                  frame "AboutAzCam" {
                    w419 = "\nWritten by Michael Lesser, University of Arizona\nSee http://www.itl.arizona.edu\nLabVIEW is copyright National Instruments, Inc."  # Written by Michael Lesser, University of Arizona See http://www.itl.arizona.edu LabVIEW is copyright National Instruments, Inc.
                    n312 = global read "AzCamGlobals.vi" "Version"() -> (w421:string)
                    n313 = Concatenate Strings("Version: " ("message"), w421, w419) -> (w418:string)
                    n314 = One Button Dialog(message=w418) -> ()  [unwired: 1 in, 1 out]
                  }
                }
              }
            }
          }
        }
      }
      frame "Exit" {
        n315 = stacked-sequence {
          frame #0 {
            # "update ConfigFile"
            n316 = stacked-sequence {
              frame #0 {
                n317 = call "FPposition.vi"("Action"=enum16{"Make string", "Decode string"}."Make string") -> ("String Out"=w425:string)  [unwired: 1 in, 2 out]
                n318 = call "SetAzCamToolParameter.vi"("Value"=w425, "Parameter"="frontpanelposition" ("key")) -> ()  [unwired: 1 out]
              }
              frame #1 {
                n319 = global read "AzCamGlobals.vi" "UserWarnings"() -> (w428:bool)
                n320 = Select(t="1" ("y"), s=w428, f="0" ("y")) -> (s? t:f=w426:string)
                n321 = call "SetAzCamToolParameter.vi"("Value"=w426, "Parameter"="UserWarnings" ("key")) -> ()  [unwired: 1 out]
              }
              frame #2 {
                n322 = global read "AzCamGlobals.vi" "Prompt4Title"() -> (w435:bool)
                n323 = Select(t="1" ("y"), s=w435, f="0" ("y")) -> (s? t:f=w431:string)
                n324 = call "SetAzCamToolParameter.vi"("Value"=w431, "Parameter"="PromptForTitle" ("key")) -> ()  [unwired: 1 out]
              }
              frame #3 {
                n325 = global read "AzCamGlobals.vi" "UseSound"() -> (w445:bool)
                n326 = Select(t="1" ("Parameter"), s=w445, f="0" ("Parameter")) -> (s? t:f=w438:string)
                n327 = global read "AzCamGlobals.vi" "ReadTemps"() -> (w440:bool)
                n328 = call "SetAzCamToolParameter.vi"("Value"=w438, "Parameter"="UseSound") -> ()  [unwired: 1 out]
                n329 = Select(t="1" ("Parameter"), s=w440, f="0" ("Parameter")) -> (s? t:f=w436:string)
                n330 = call "SetAzCamToolParameter.vi"("Value"=w436, "Parameter"="ReadTemperatures") -> ()  [unwired: 1 out]
              }
              frame #4 {
                n331 = call "SavePars.vi"() -> ()  [unwired: 1 in, 1 out]
              }
            }
          }
          frame #1 {
            n332 = flat-sequence {
              frame #0 {
                n333 = global read "AzCamGlobals.vi" "ShutDown"() -> (w446:bool)
                n334 = case shown="True" w446 {
                  frame False {
                  }
                  frame True {
                    n335 = call "ServerCommand.vi"("Command"="exitazcam") -> ()  [unwired: 2 out]
                  }
                }
              }
              frame #1 {
                n336 = global write "AzCamGlobals.vi" "SocketOpen"(FALSE ("SocketOpen?")) -> ()
                n337 = global read "AzCamGlobals.vi" "ConnectionID"() -> (w449:refnum<k5>)
                n338 = TCP Close Connection(connection ID=w449) -> ()  [unwired: 2 in, 2 out]
              }
            }
          }
          frame #2 {
            # "close AzCamTool"
            n339 = property class="App"() -> ("Application:Kind"=w452:T6)  [unwired: 2 in, 2 out]
            n340 = Equal?(x=w452, y=T6."Run Time System" ("Application:Kind")) -> (x = y?=w450:bool)
            n341 = case shown="False" w450 {
              selector: w450 -> [_ w453]
              frame False {
                n342 = Stop() -> ()  [unwired: 1 in]
              }
              frame True {
                n343 = Quit LabVIEW(quit? (T)=w453) -> ()
              }
            }
          }
        }
      }
      frame "Quit" {
        n344 = flat-sequence {
          frame #0 {
            n345 = local write "StatusBar"("Shutting down..." ("message")) -> ()
            n346 = Wait (ms)(milliseconds to wait=u32 1000) -> ()  [unwired: 1 out]
          }
          frame #1 {
            n347 = property class="App"() -> ("Application:Kind"=w457:T6)  [unwired: 2 in, 2 out]
            n348 = Equal?(x=w457, y=T6."Run Time System" ("Application:Kind")) -> (x = y?=w459:bool)
            n349 = case shown="False" w459 {
              selector: w459 -> [_ w460]
              frame False {
                n350 = Stop() -> ()  [unwired: 1 in]
              }
              frame True {
                n351 = Quit LabVIEW(quit? (T)=w460) -> ()
              }
            }
          }
        }
      }
    }
  }
